vi "FireMotor.vi"   [LabVIEW 2012]
uses:
  StateMachineEnum.ctl
  Robot Global Data.vi
types:
  T1 = typedef "StateMachineEnum.ctl" = enum16{"Init", "Idle", "Start", "Do", "Stop"}
  T2 = typedef "WPI_MotorControlDeviceRef.ctl" = cluster{"DeviceStatus":errorcluster, "Type":enum16{"PWM", "CAN"}, "PWM":cluster{"Digital Module":T3, "PWM Channel":T4, "DeadBand":T5}, "CAN":cluster{"Device Number":u8, "Control Mode":T6, "Semaphore":T7, "Max Vout":dbl}, "Invert":bool, "TransformRef":T8, "InvTransformRef":T8}
  T3 = typedef "FPGA_TypedefDigitalModule.ctl" = enum16{"Digital Module 1", "Digital Module 2"}
  T4 = typedef "FPGA_DIOPWMChannel.ctl" = enum8{"PWM 1", "PWM 2", "PWM 3", "PWM 4", "PWM 5", "PWM 6", "PWM 7", "PWM 8", "PWM 9", "PWM 10", "Invalid"}
  T5 = typedef "WPI_PWMDeadband.ctl" = cluster{"Name":string, "maxPositivePwm":i32, "minPositivePwm":i32, "centerPwm":i32, "maxNegativePwm":i32, "minNegativePwm":i32, "angularRange":u16}
  T6 = typedef "WPI_CANJaguar_ControlMode.ctl" = enum8{"Percent VBus", "Current", "Speed", "Position", "Voltage"}
  T7 = typedef "Semaphore RefNum" = refnum<k1>
  T8 = typedef "WPI_PWMTransform_ConPane.ctl" = refnum<vi>
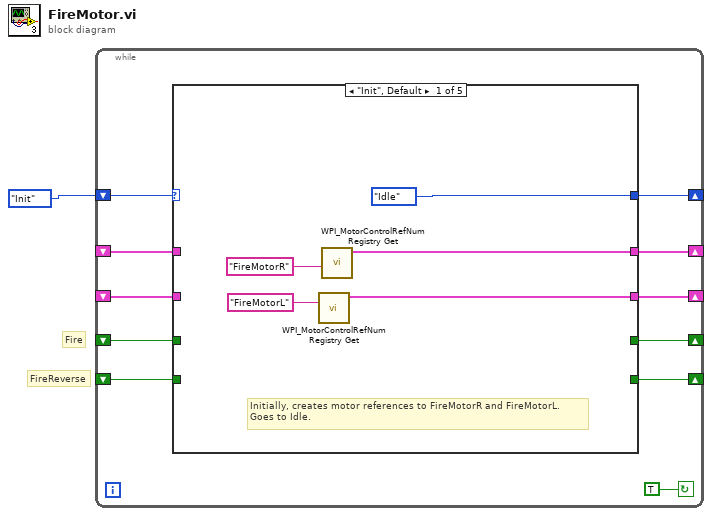
[diagram p0: block diagram]
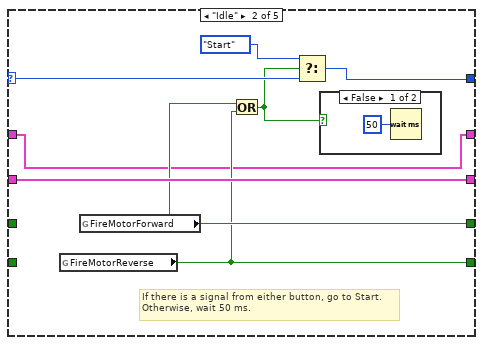
[diagram p2: hidden frame]
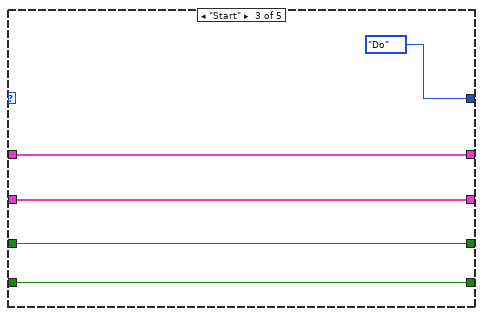
[diagram p4: hidden frame]
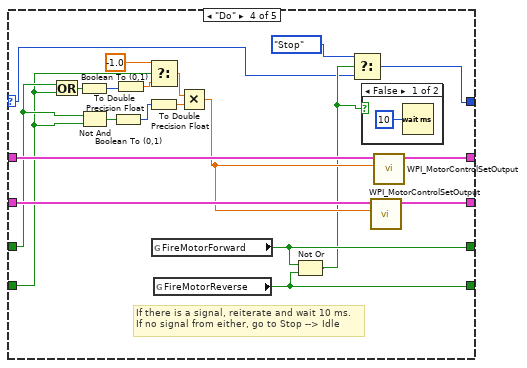
[diagram p5: hidden frame]
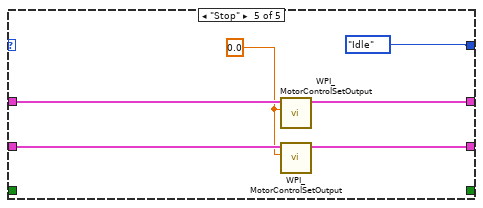
[diagram p7: hidden frame]
diagram:
  # "FireReverse"
  # "Fire"
  n1 = while {
    shift-right: [w2] -> _
    shift-left: StateMachineEnum."Init" ("State") -> [w7]
    shift-right: [w12] -> _
    shift-left: _ -> [w9]
    shift-right: [w11] -> _
    shift-left: _ -> [w8]
    shift-right: [w5] -> _
    shift-left: _ -> [w3]
    shift-right: [w6] -> _
    shift-left: _ -> [w4]
    stop <- TRUE continue-if-true
    n2 = case shown="\"Init\", Default" w7 {
      selector: w7 -> [_ w23 _ w32 _]
      tunnel: [StateMachineEnum."Idle" ("State") w19 StateMachineEnum."Do" ("State") w47 StateMachineEnum."Idle" ("State")] -> w2
      tunnel: [w14 w20 w28 w49 w56] -> w12
      tunnel: [w13 w24 w27 w51 w57] -> w11
      tunnel: w9 -> [_ w20 w28 w50 w55]
      tunnel: w8 -> [_ w24 w27 w52 w58]
      tunnel: [_ w21 w29 w34 _] -> w6
      tunnel: [_ w22 w30 w35 _] -> w5
      tunnel: w4 -> [_ _ w29 w43 _]
      tunnel: w3 -> [_ _ w30 w44 _]
      frame "Init", Default {
        # "Initially, creates motor references to FireMotorR and FireMotorL.\nGoes to Idle."
        n3 = call <vilib>:"WPI_MotorControlRefNum Registry Get.vi"("refnum name"="FireMotorL") -> ("MotorControlDevRef"=w13:T2)  [unwired: 9 in, 1 out]
        n4 = call <vilib>:"WPI_MotorControlRefNum Registry Get.vi"("refnum name"="FireMotorR") -> ("MotorControlDevRef"=w14:T2)  [unwired: 9 in, 1 out]
      }
      frame "Idle" {
        # "If there is a signal from either button, go to Start.\nOtherwise, wait 50 ms."
        n5 = global read "Robot Global Data.vi" "FireMotorReverse"() -> (w21:bool)
        n6 = global read "Robot Global Data.vi" "FireMotorForward"() -> (w22:bool)
        n7 = Or(x=w22, y=w21) -> (x .or. y?=w18:bool)
        n8 = Select(t=StateMachineEnum."Start" ("State"), s=w18, f=w23) -> (s? t:f=w19:T1)
        n9 = case shown="False" w18 {
          frame False {
            n10 = Wait (ms)(milliseconds to wait=u32 50) -> ()  [unwired: 1 out]
          }
          frame True {
          }
        }
      }
      frame "Start" {
      }
      frame "Do" {
        # "If there is a signal, reiterate and wait 10 ms.\nIf no signal from either, go to Stop --> Idle"
        n11 = Or(x=w44, y=w43) -> (x .or. y?=w46:bool)
        n12 = Boolean To (0,1)(Boolean=w46) -> (0, 1=w45:i16)
        n13 = Not And(1:w43, 2:w44) -> (0:w42:bool)
        n14 = Boolean To (0,1)(Boolean=w42) -> (0, 1=w40:i16)
        n15 = To Double Precision Float(number=w45) -> (double precision float=w37:dbl)
        n16 = Select(t=-1.0, s=w43, f=w37) -> (s? t:f=w41:dbl)
        n17 = To Double Precision Float(number=w40) -> (double precision float=w38:dbl)
        n18 = global read "Robot Global Data.vi" "FireMotorForward"() -> (w35:bool)
        n19 = global read "Robot Global Data.vi" "FireMotorReverse"() -> (w34:bool)
        n20 = Multiply(x=w41, y=w38) -> (x*y=w39:dbl)
        n21 = Not Or(1:w34, 2:w35) -> (0:w33:bool)
        n22 = Select(t=StateMachineEnum."Stop" ("State"), s=w33, f=w32) -> (s? t:f=w47:T1)
        n23 = case shown="False" w33 {
          frame False {
            n24 = Wait (ms)(milliseconds to wait=u32 10) -> ()  [unwired: 1 out]
          }
          frame True {
          }
        }
        n25 = call <vilib>:"WPI_MotorControlSetOutput.vi"("Output"=w39, "MotorControlDevRef"=w52) -> ("MotorControlDevRef"=w51:T2)  [unwired: 7 in, 2 out]
        n26 = call <vilib>:"WPI_MotorControlSetOutput.vi"("Output"=w39, "MotorControlDevRef"=w50) -> ("MotorControlDevRef"=w49:T2)  [unwired: 7 in, 2 out]
      }
      frame "Stop" {
        w54 = 0.0
        n27 = call <vilib>:"WPI_MotorControlSetOutput.vi"("Output"=w54, "MotorControlDevRef"=w55) -> ("MotorControlDevRef"=w56:T2)  [unwired: 7 in, 2 out]
        n28 = call <vilib>:"WPI_MotorControlSetOutput.vi"("Output"=w54, "MotorControlDevRef"=w58) -> ("MotorControlDevRef"=w57:T2)  [unwired: 7 in, 2 out]
      }
    }
  }
